vi "create-style_css.vi"(8 "error in (no error)":errorcluster, 11 "path to .css file":path) -> (0 "error out":errorcluster, 3 "path":path)   [LabVIEW 2014]
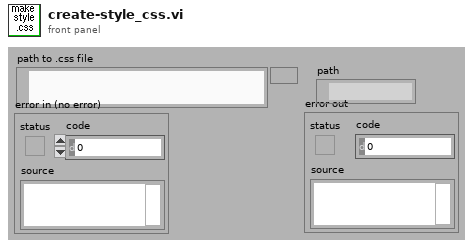
[diagram p1: front panel]
types:
  T1 = enum16{"open", "replace", "create", "open or create", "replace or create", "replace or create with confirmation"}
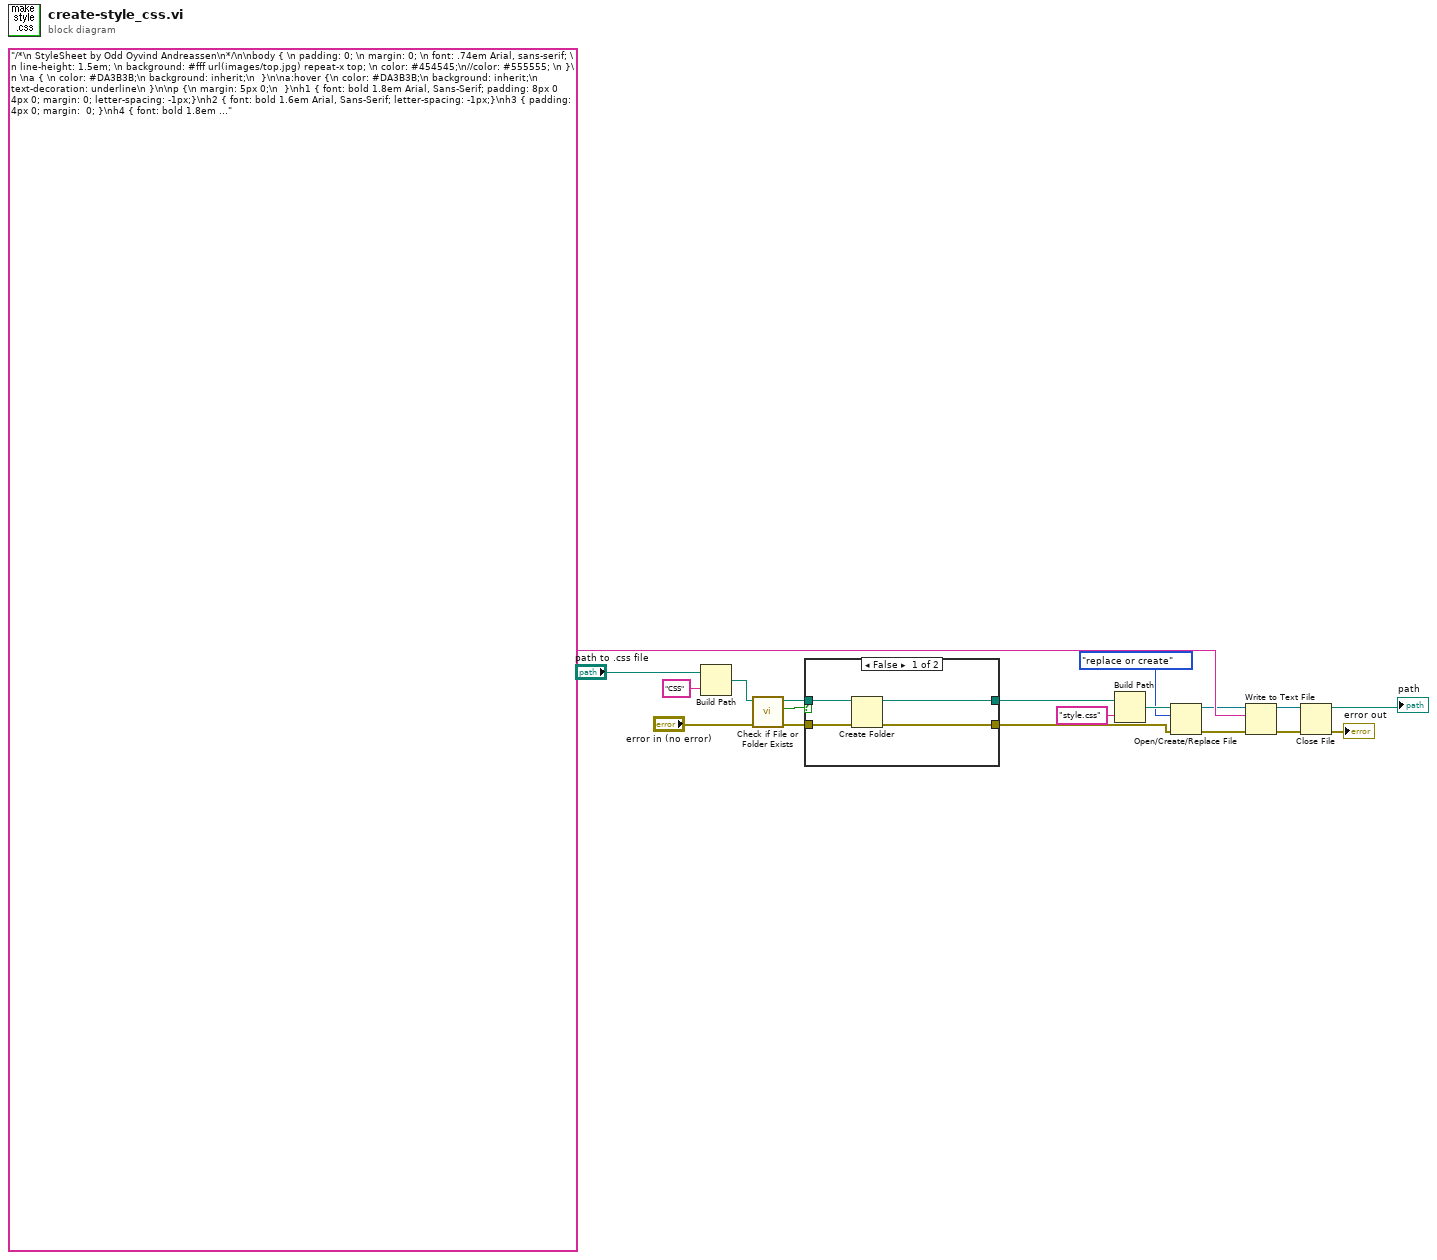
[diagram p0: block diagram]
diagram:
  n1 = Build Path(base path="path to .css file", name or relative path="CSS") -> (appended path=w3:path)
  n2 = call <vilib>:"Check if File or Folder Exists.vi"("error in (no error)"="error in (no error)", "path"=w3) -> ("error out"=w13:errorcluster, "file or folder exists?"=w14:bool, "dup path"=w15:path)  [unwired: 7 out]
  n3 = case shown="False" w14 {
    tunnel: w15 -> [w23 w25]
    tunnel: w13 -> [w22 w24]
    tunnel: [w21 w25] -> w12
    tunnel: [w20 w24] -> w8
    frame False {
      n4 = Create Folder(path (use dialog)=w23, error in=w22) -> (created path=w21:path, error out=w20:errorcluster)  [unwired: 2 out]
    }
    frame True {
    }
  }
  n5 = Build Path(base path=w12, name or relative path="style.css") -> (appended path=w11:path)
  n6 = Open/Create/Replace File(file path (use dialog)=w11, error in=w8, operation (0:open)=T1."replace or create") -> (refnum out=w10:refnum<file>, error out=w7:errorcluster)  [unwired: 4 out]
  n7 = Write to Text File(file (use dialog)=w10, text="/*\n StyleSheet by Odd Oyvind Andreassen\n*/\n\nbody { \n padding: 0; \n margin: 0; \n font: .74em Arial, sans-serif; \n line-height: 1.5em; \n background: #fff url(images/top.jpg) repeat-x top; \n color: #454545;\n//color: #555555; \n }\n \na { \n color: #DA3B3B;\n background: inherit;\n  }\n\na:hover {\n color: #DA3B3B;\n background: inherit;\n text-decoration: underline\n }\n\np {\n margin: 5px 0;\n  }\nh1 { font: bold 1.8em Arial, Sans-Serif; padding: 8px 0 4px 0; margin: 0; letter-spacing: -1px;}\nh2 { font: bold 1.6em Arial, Sans-Serif; letter-spacing: -1px;}\nh3 { padding: 4px 0; margin:  0; }\nh4 { font: bold 1.8em Arial, Sans-Serif; padding: 8px 0 4px 0; margin: 0; letter-spacing: -1px; color: #959595;}\nh5{ font: bold 1.6em Arial, Sans-Serif; letter-spacing: -1px; color: #959595;}\nul { margin: 0; padding : 0; list-style: none; }\nimg { border: 0; }\nhr { height: 1px; border-style: none; color: #d0d0d0; background-color: #C0C0C0; margin: 10px 0; }\n\n/* to center all items below header */\n.content {\n margin: 0px auto;\n width: 900px;\n }\n/* Red Box Header */\n#wrap { \n margin: 30px auto;\n width: 900px;\n height: 20px; \n }\n \n   #wrap #pic {\n float: left;\n background: #FF0000 url(images/main800x40.jpg) no-repeat;\n height: 40px;\n width: 800px;\n overflow: hidden\n }\n\n   #wrap #pic #slogan { \n float: left; \n padding: 1px 1px 1px 30px;\n text-align: left \n }\n\n   #wrap #pic #slogan h1 {\n font: bold 2.0em Arial, Sans-Serif;\n color: #FFF;\n letter-spacing: 0px;\n margin:0\n }\n\n   #wrap #pic #slogan h2 {\n font: 1.5em Arial, Sans-Serif;\n color: #FFF;\n letter-spacing: 0px;\n margin: 0;\n }   \n\n   #wrap #pic #slogan a {\n color: #FFF;\n }", error in=w7) -> (refnum out=w18:refnum<file>, error out=w19:errorcluster)  [unwired: 2 out]
  n8 = Close File(refnum=w18, error in=w19) -> (path=→"path":path, error out=→"error out":errorcluster)
